vi "EditDisconFile.vi"(4 "To VS_ControlMode":T1(ring), 5 "Append":string, 6 "Edit DISCON":bool, 8 "From VS_ControlMode":T1(ring), 9 "path":path) -> (2 "result string":string, 3 "data":string)   [LabVIEW 2018]
panel:
  in  "DISCON.IN Contents":string
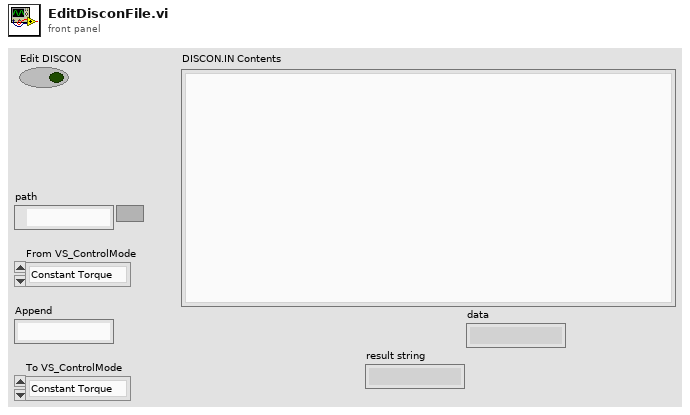
[diagram p1: front panel]
types:
  T1 = enum16{"Constant Torque", "Constant Power", "PI Control"}
  T2 = enum16{"open", "replace", "create", "open or create", "replace or create", "replace or create with confirmation"}
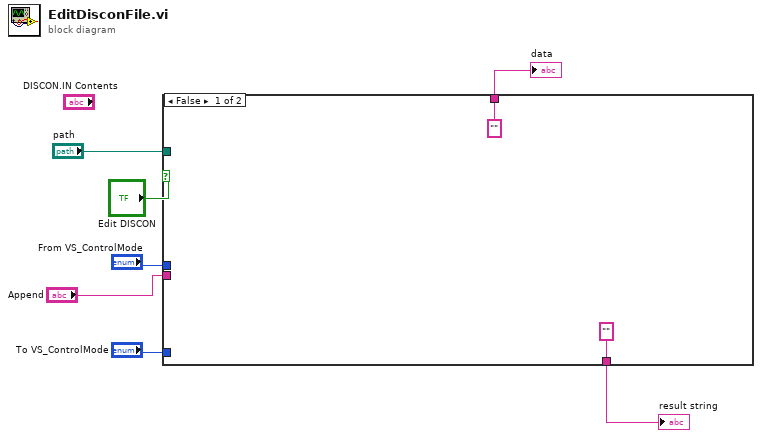
[diagram p0: block diagram]
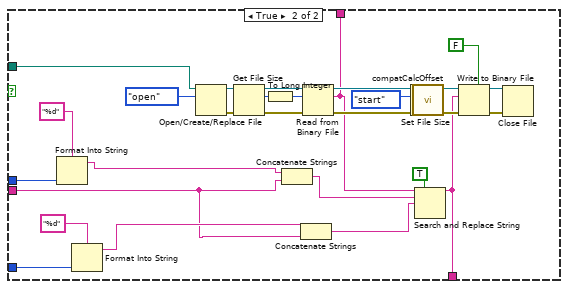
[diagram p2: hidden frame]
diagram:
  n1 = case shown="False" "Edit DISCON" {
    tunnel: "To VS_ControlMode" -> [_ w22]
    tunnel: "From VS_ControlMode" -> [_ w18]
    tunnel: "Append" -> [_ w13]
    tunnel: "path" -> [_ w12]
    tunnel: ["" w11] -> w2
    tunnel: ["" ("result string") w10] -> w1
    frame False {
    }
    frame True {
      n2 = Format Into String(format string="%d", w18) -> (resulting string=w17:string)  [unwired: 2 in, 1 out]
      n3 = Format Into String(format string="%d", w22) -> (resulting string=w16:string)  [unwired: 2 in, 1 out]
      n4 = Open/Create/Replace File(file path (use dialog)=w12, operation (0:open)=T2."open") -> (refnum out=w40:refnum<file>, error out=w39:errorcluster)  [unwired: 4 in, 1 out]
      n5 = Get File Size(file=w40, error in=w39) -> (refnum out=w38:refnum<file>, size (in bytes)=w23:i64, 0:w37:errorcluster)
      n6 = To Long Integer(number=w23) -> (32bit integer=w36:i32)
      n7 = Concatenate Strings(w17, w13) -> (w15:string)
      n8 = Concatenate Strings(w16, w13) -> (w14:string)
      n9 = Read from Binary File(8:w37, 10:w36, 11:w38) -> (0:w30:errorcluster, 2:w11:string, 3:w28:refnum<file>)  [unwired: 3 in, 1 out]
      n10 = call <vilib>:"compatCalcOffset.vi"("error in"=w30, "pos mode (0:1)"=enum16{"start", "end", "current"}."start", "refnum"=w28) -> ("error out"=w27:errorcluster, "offset"=w26:i32, "dup refnum"=w25:refnum<file>)  [unwired: 6 in]
      n11 = Set File Size(4:w27, 6:w26, 7:w25) -> (0:w31:errorcluster, 3:w32:refnum<file>)
      n12 = Search and Replace String(replace all?=TRUE ("replace all? (F)"), input string=w11, search string=w15, replace string=w14) -> (result string=w10:string)  [unwired: 4 in, 3 out]
      n13 = Write to Binary File(file (use dialog)=w32, data=w10, error in=w31, 5:FALSE ("prepend array or string size? (T)")) -> (refnum out=w33:refnum<file>, error out=w34:errorcluster)  [unwired: 2 in, 1 out]
      n14 = Close File(refnum=w33, error in=w34) -> ()  [unwired: 2 out]
    }
  }
  "data" <- w2
  "result string" <- w1
